vi "DBM DB Insert.vi"(5 "Query info":T2, 6 "Value":string[][](array[string]), 7 "Slide 입력":refnum<vi>, 8 "에러 입력":errorcluster caption="에러 입력(에러 없음)", 10 "COMMAND":T3, 11 "참조 번호 입력":T1) -> (0 "에러 출력":errorcluster, 3 "참조 번호 출력":T1)   [LabVIEW 2020]
uses:
  Controls/Cmd_Write Query.ctl
  Controls/Clst_Query Info.ctl
  <vilib>/addons/database/Connection.llb/Conn ObjectReference.ctl
  <vilib>/addons/database/NI_Database_API.lvlib
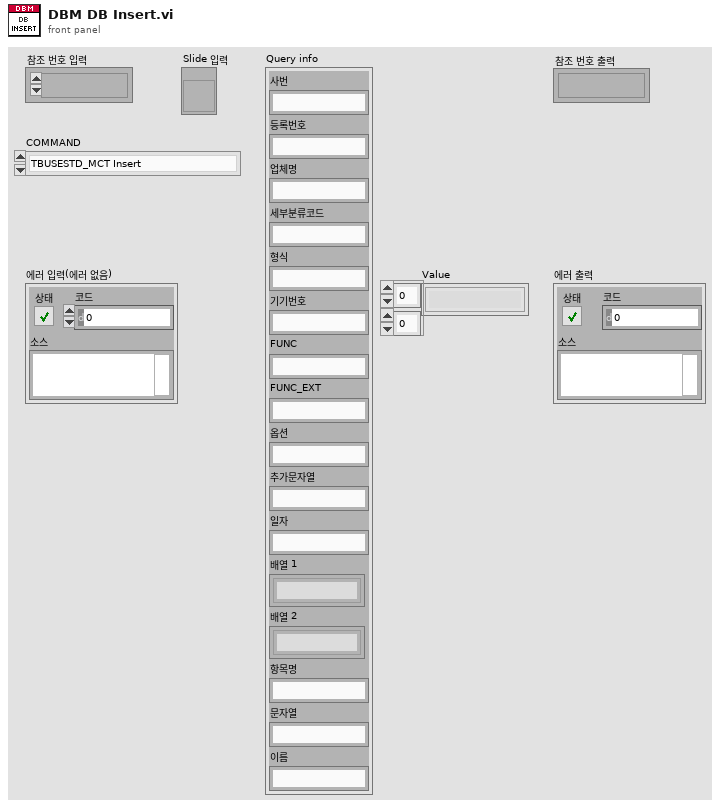
[diagram p1: front panel]
types:
  T1 = typedef "NI_Database_API.lvlib/Conn ObjectReference.ctl" = refnum<k1>
  T2 = typedef "Clst_Query Info.ctl" = cluster{"사번":string, "등록번호":string, "업체명":string, "세부분류코드":string, "형식":string, "기기번호":string, "FUNC":string, "FUNC_EXT":string, "옵션":string, "추가문자열":string, "일자":string, "배열 1":string[], "배열 2":string[], "항목명":string, "문자열":string, "이름":string}
  T3 = typedef "Cmd_Write Query.ctl" = enum16{"TBUSESTD_MCT Insert", "TBUSESTD_MCT Delete", "TBCALSTD_MCT_TEMP Insert", "TBCALSTD_MCT_TEMP Delete", "TBCALSTD_MCT Insert", "TBCALSTD_MCT Delete", "TBCALSTD_MCT_BACK Insert", "TBCALSTD_MCT_BACK Delete", "TBCALPROC_MCT Insert", "TBCALPROC_MCT Delete", "TBCALPROC_MCT_TEMP Insert", "TBCALPROC_MCT_TEMP Delete", "TBCALCMC_MCT Insert", "TBCALCMC_MCT Delete", "TBCALFUNC_MCT Insert", "TBCALFUNC_MCT Delete", "TBCALNAME_MCT Insert", "TBCALNAME_MCT Delete", "TBSTDNAME_MCT Insert", "TBSTDNAME_MCT Delete", "TBCALSPEC_MCT Insert", "TBCALSPEC_MCT Delete", "TBCALSTD_MCT NOTUSE update", "TBCALSPEC_MCT update", "TBMCTVERMAN update"}
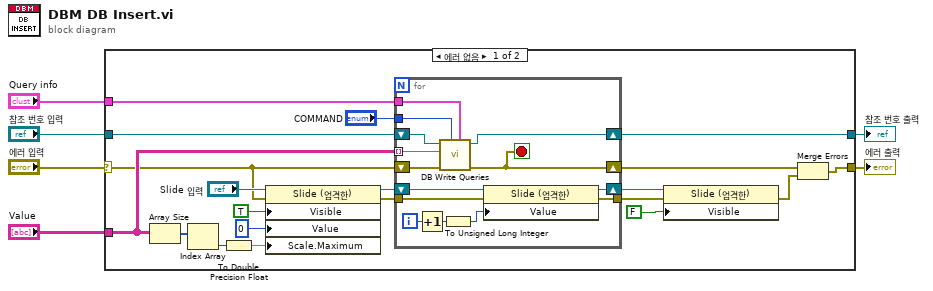
[diagram p0: block diagram]
diagram:
  n1 = case shown="에러 없음" "에러 입력" {
    selector: "에러 입력" -> [w10 w41]
    tunnel: "참조 번호 입력" -> [w26 w42]
    tunnel: [w25 w42] -> w3
    tunnel: "Value" -> [w23 _]
    tunnel: [w14 w41] -> w2
    tunnel: "Query info" -> [w16 _]
    frame No Error {
      n2 = Array Size(array=w23) -> (size(s)=w22:i32[])
      n3 = Index Array(array=w22) -> (element=w21:i32)  [unwired: 1 in]
      n4 = To Double Precision Float(number=w21) -> (double precision float=w11:dbl)
      n5 = property on="프로퍼티 노드" class="Slide (엄격한)"(reference="Slide 입력", error in=w10, "Visible"=TRUE ("보이기"), "Value"=u32 0 ("값"), "Scale.Maximum"=w11) -> (reference out=w24:refnum<vi>, error out=w9:errorcluster)
      n6 = for {
        tunnel: "COMMAND" -> [w38]
        shift-right: [w39] -> w25
        shift-left: w26 -> [w40]
        tunnel: w23 -> [w37] mode=indexing
        shift-right: [w32] -> w19
        shift-left: w24 -> [w33]
        tunnel: w16 -> [w31]
        shift-right: [w29] -> w8
        shift-left: w10 -> [w30]
        tunnel: w9 -> [w28]
        tunnel: [w27] -> w7
        i -> [w36]
        stop <- w29 stop-if-true
        n7 = Increment(x=w36) -> (x+1=w34:i32)
        n8 = call "DB Write Queries.vi"("Query info"=w31, "COMMAND"=w38, "에러 입력(에러 없음)"=w30, "DATA IN"=w37, "참조 번호 입력"=w40) -> ("에러 출력"=w29:errorcluster, "참조 번호 출력"=w39:T1)  [unwired: 5 in]
        n9 = To Unsigned Long Integer(number=w34) -> (unsigned 32bit integer=w35:u32)
        n10 = property on="프로퍼티 노드" class="Slide (엄격한)"(reference=w33, error in=w28, "Value"=w35) -> (reference out=w32:refnum<vi>, error out=w27:errorcluster)
      }
      n11 = property on="프로퍼티 노드" class="Slide (엄격한)"(reference=w19, error in=w7, "Visible"=FALSE ("보이기")) -> (error out=w18:errorcluster)  [unwired: 1 out]
      n12 = Merge Errors(w8, w18) -> (w14:errorcluster)
    }
    frame Error {
    }
  }
  "참조 번호 출력" <- w3
  "에러 출력" <- w2
